vi "LabVIEW NPOI Project.vi"   [LabVIEW 2017]
uses:
  <vilib>/Platform/browser.llb/Open URL in Default Browser (string).vi
panel:
  # "Opening LabVIEW NPOI Project Page..."
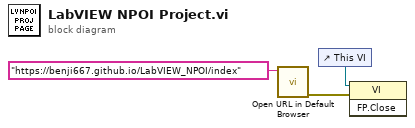
[diagram p0: block diagram]
diagram:
  n1 = call-poly <vilib>:"Open URL in Default Browser.vi"("URL"="https://benji667.github.io/LabVIEW_NPOI/index") -> ("error out"=w3:errorcluster)  [unwired: 5 in, 1 out]
  n2 = control-ref of="This VI"() -> (w2:refnum<vi>)
  n3 = invoke class="VI" method="FP.Close"(reference=w2, error in=w3) -> ()  [unwired: 1 in, 3 out]
